vi "setPrecisionMulti.vi"(9 "Precision":u32, 10 "Numbers":dbl[](array[numeric])) -> (2 "Rounded Numbers":dbl[](array[numeric]))   [LabVIEW 2011]
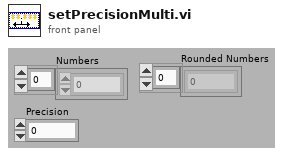
[diagram p1: front panel]
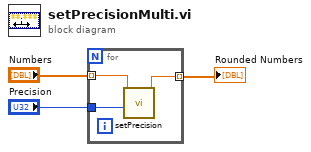
[diagram p0: block diagram]
diagram:
  n1 = for {
    tunnel: "Precision" -> [w6]
    tunnel: "Numbers" -> [w5] mode=indexing
    tunnel: [w4] -> w1 mode=indexing
    n2 = call "setPrecision.vi"("Precision"=w6, "Number"=w5) -> ("Rounded Number"=w4:dbl)  [unwired: 9 in]
  }
  "Rounded Numbers" <- w1
